vi "Find All Accessors.vi"(6 "Mouse Position":T1, 7 "User VI Ref":refnum<vi>, 8 "Is Multi-select?":bool, 9 "Remaining Items":refnum<vi>[](array[refnum]), 10 "Affected Items":T8, 11 "Menu Refnum":refnum<k9>) -> (3 "Menu Items To Add":T2[](array[typedef]))   [LabVIEW 2020]
doc: "This VI is part of a plug-in for modifying the LabVIEW shortcut menus. This is the builder VI which is called when the shortcut menu is built. It tells LabVIEW which shortcut menu items to add to the menu."
uses:
  <resource>/plugins/PopupMenus/support/Shortcut Menu Item Definition.ctl
  <resource>/plugins/PopupMenus/support/Transaction Control.ctl
  <resource>/plugins/PopupMenus/support/Position In Menu.ctl
  <resource>/plugins/PopupMenus/support/Relative Position.ctl
  <resource>/plugins/PopupMenus/support/Checkmark Status.ctl
  <resource>/plugins/PopupMenus/support/Enabled Menu Item Status.ctl
  Find All Accessors.ctl
  <vilib>/Utility/miscctls.llb/LVPositionTypeDef.ctl
panel:
  # "Rules a popup plug-in must follow:\n* This VI's file name must match the file name of the LLB -- only the file extensions should be different.\n* This VI must have debugging disabled or it will be ignored as a plug-in.\n* For all menu items, \"tag suffix + file name of this VI\" must be less than 240 characters.\n* You can disconnect the \"Affected Items\" from the typedef to make the plug-in load faster. The typedef is only there to assist you in keeping this VI and the execution VI using to the same type.\n* All controls on this panel except \"Affected Items\" are locked to prevent accidental edits. Do not change the types or the names of controls other than the elements inside the \"Affected Items\" cluster.\n* See Context Help for more information on the individual controls."
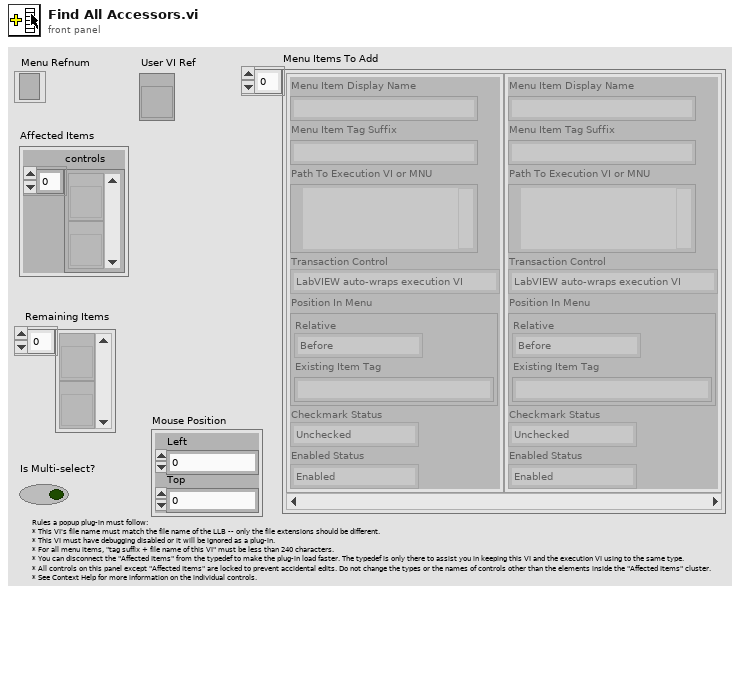
[diagram p1: front panel]
types:
  T1 = typedef "LVPositionTypeDef.ctl" = cluster{"Left":i32, "Top":i32}
  T2 = typedef "Shortcut Menu Item Definition.ctl" = cluster{"Menu Item Display Name":string, "Menu Item Tag Suffix":string, "Path To Execution VI or MNU":path, "Transaction Control":T3, "Position In Menu":T4, "Checkmark Status":T6, "Enabled Status":T7}
  T3 = typedef "Transaction Control.ctl" = enum8{"LabVIEW auto-wraps execution VI", "Execution VI will define if needed"}
  T4 = typedef "Position In Menu.ctl" = cluster{"Relative":T5, "Existing Item Tag":string}
  T5 = typedef "Relative Position.ctl" = enum8{"Before", "Instead of", "After", "Into Submenu"}
  T6 = typedef "Checkmark Status.ctl" = enum8{"Unchecked", "Checked"}
  T7 = typedef "Enabled Menu Item Status.ctl" = enum8{"Enabled", "Disabled"}
  T8 = typedef "Find All Accessors.ctl" = cluster{"controls":refnum<vi>[]}
  T9 = enum32{"not a control VI", "control", "typedef", "strict typedef"}
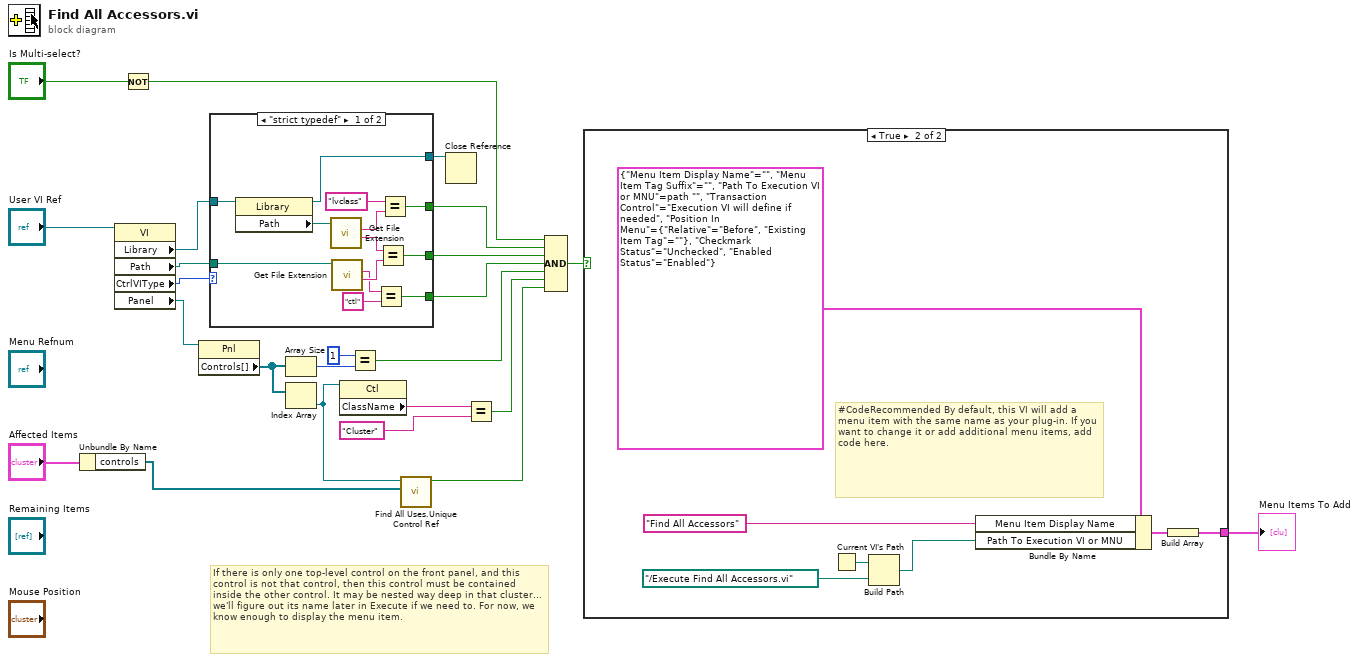
[diagram p0: block diagram]
diagram:
  # "If there is only one top-level control on the front panel, and this control is not that control, then this control must be contained inside the other control. It may be nested way deep in that cluster... we'll figure out its name later in Execute if we need to. For now, we know enough to display the menu item."
  n1 = Unbundle By Name("Affected Items") -> ("controls"=w3:refnum<vi>[])
  n2 = property class="VI"(reference="User VI Ref") -> ("Library"=w19:refnum<vi>, "Path"=w20:path, "CtrlVIType"=w21:T9, "Panel"=w17:refnum<vi>)  [unwired: 1 in, 2 out]
  n3 = Not(x="Is Multi-select?") -> (.not. x?=w9:bool)
  n4 = property class="Pnl"(reference=w17) -> ("Controls[]"=w14:refnum<vi>[])  [unwired: 1 in, 2 out]
  n5 = case shown="\"strict typedef\"" w21 {
    tunnel: w20 -> [w35 _]
    tunnel: w19 -> [w37 w38]
    tunnel: [w32 _] -> w7
    tunnel: [w29 _] -> w8
    tunnel: [w26 _] -> w5
    tunnel: [w25 w38] -> w10
    frame "strict typedef" {
      n6 = property class="Library"(reference=w37) -> (reference out=w25:refnum<vi>, "Path"=w36:path)  [unwired: 1 in, 1 out]
      n7 = call <vilib>:"Get File Extension.vi"("file"=w36) -> ("filename without extension"=w34:string, "lowercase file extension"=w30:string)  [unwired: 6 in, 3 out]
      n8 = call <vilib>:"Get File Extension.vi"("file"=w35) -> ("filename without extension"=w33:string, "lowercase file extension"=w28:string)  [unwired: 6 in, 3 out]
      n9 = Equal?(x=w28, y="ctl") -> (x = y?=w26:bool)
      n10 = Equal?(x=w34, y=w33) -> (x = y?=w32:bool)
      n11 = Equal?(x="lvclass", y=w30) -> (x = y?=w29:bool)
    }
    frame Default {
    }
  }
  n12 = Array Size(array=w14) -> (size(s)=w16:i32)
  n13 = Index Array(array=w14) -> (element=w2:refnum<vi>)  [unwired: 1 in]
  n14 = property class="Ctl"(reference=w2) -> ("ClassName"=w13:string)  [unwired: 1 in, 2 out]
  n15 = Equal?(x=1, y=w16) -> (x = y?=w4:bool)
  n16 = call "Find All Uses.Unique Control Ref.vi"("controls"=w3, "top cluster"=w2) -> ("unique?"=w1:bool)  [unwired: 8 in, 1 out]
  n17 = Close Reference(reference=w10) -> ()  [unwired: 1 in, 1 out]
  n18 = Equal?(x=w13, y="Cluster" ("Class Name")) -> (x = y?=w6:bool)
  n19 = Compound Arithmetic op=AND(w9, w8, w7, w5, w4, w6, w1) -> (w11:bool)
  n20 = case shown="True" w11 {
    tunnel: [_ w41] -> w24
    frame False {
    }
    frame True {
      # "#CodeRecommended By default, this VI will add a menu item with the same name as your plug-in. If you want to change it or add additional menu items, add code here."
      n21 = Current VI's Path() -> (path=w40:path)
      n22 = Build Path(base path=w40, name or relative path=path "../Execute Find All Accessors.vi" ("execute path")) -> (appended path=w44:path)
      n23 = Bundle By Name(cluster=T2 {"Menu Item Display Name"="", "Menu Item Tag Suffix"="", "Path To Execution VI or MNU"=path "", "Transaction Control"=enum."Execution VI will define if needed", "Position In Menu"={"Relative"=enum."Before", "Existing Item Tag"=""}, "Checkmark Status"=enum."Unchecked", "Enabled Status"=enum."Enabled"} ("Cluster"), "Menu Item Display Name"="Find All Accessors", "Path To Execution VI or MNU"=w44) -> (w42:T2)
      n24 = Build Array(w42) -> (w41:T2[])
    }
  }
  "Menu Items To Add" <- w24
